vi "Close.vi"(8 "error in (no error)":errorcluster, 11 "RMX4120 in":refnum<class "RMX4120.lvclass">) -> (0 "error out":errorcluster, 3 "RMX4120 out":refnum<class "RMX4120.lvclass">)   [LabVIEW 2023, in "RMX4120.lvclass"]
uses:
  RMX4120.lvclass
  RMXPowerSupply.lvclass
  RMX4120.lvclass/RMX4120.ctl
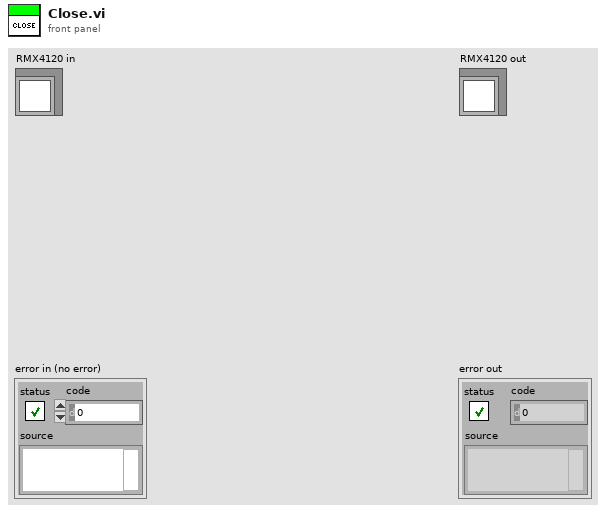
[diagram p1: front panel]
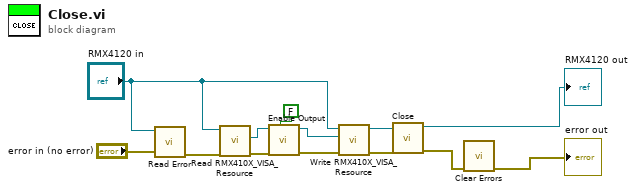
[diagram p0: block diagram]
diagram:
  n1 = call-dynamic "Read Error.vi"("error in (no error)"="error in (no error)", "RMXPowerSupply in"="RMX4120 in") -> ("error out"=w11:errorcluster)  [unwired: 7 in, 2 out]
  n2 = call-dynamic "Read RMX410X_VISA_Resource.vi"("error in (no error)"=w11, "RMXPowerSupply in"="RMX4120 in") -> ("error out"=w9:errorcluster, "RMX410X_VISA_Resource"=w8:refnum<visa-resource-name>)  [unwired: 7 in, 1 out]
  n3 = call "Enable Output.vi"("Enable Output (F: Disable)"=FALSE, "error in (no error)"=w9, "VISA resource name"=w8) -> ("error out"=w7:errorcluster, "VISA resource name out"=w4:refnum<visa-resource-name>)  [unwired: 7 in]
  n4 = call-dynamic "Write RMX410X_VISA_Resource.vi"("error in (no error)"=w7, "RMX410X_VISA_Resource"=w4, "RMXPowerSupply in"="RMX4120 in") -> ("error out"=w6:errorcluster, "RMXPowerSupply out"=w5:refnum<class "RMX4120.lvclass">)  [unwired: 7 in]
  n5 = call-parent "Close.vi"("error in (no error)"=w6, "RMXPowerSupply in"=w5) -> ("error out"=w3:errorcluster, "RMXPowerSupply out"=→"RMX4120 out":refnum<class "RMX4120.lvclass">)  [unwired: 8 in]
  n6 = call <vilib>:"Clear Errors.vi"("error in (no error)"=w3) -> ("error out"=→"error out":errorcluster)  [unwired: 5 in, 1 out]
